vi "writeI32.vi"(8 "error in (no error)":errorcluster, 10 "Input":i32, 11 "ModbusBuffer in":refnum<class "ModbusBufferBuilder.lvclass">) -> (0 "error out":errorcluster, 3 "ModbusBuffer out":refnum<class "ModbusBufferBuilder.lvclass">)   [LabVIEW 2016, in "ModbusBufferBuilder.lvclass"]
uses:
  ModbusBufferBuilder.lvclass
  ModbusBufferBuilder.lvclass/ModbusBufferBuilder.ctl
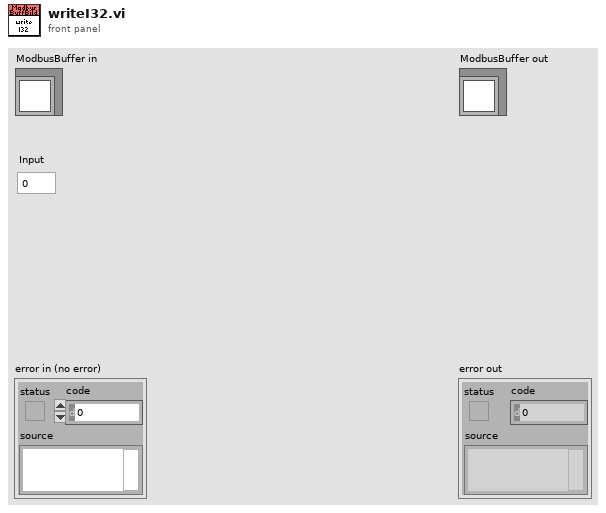
[diagram p1: front panel]
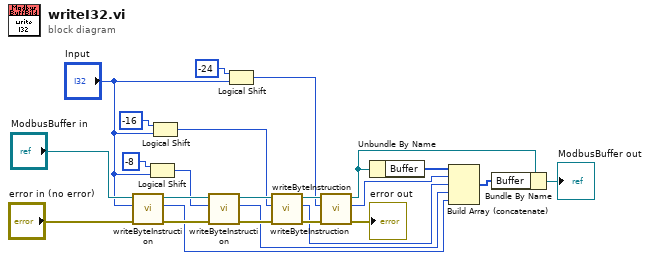
[diagram p0: block diagram]
diagram:
  n1 = call "writeByteInstruction.vi"("error in (no error)"="error in (no error)", "Input"="Input", "ModbusBuffer in"="ModbusBuffer in") -> ("error out"=w12:errorcluster, "Output"=w1:u16, "ModbusBuffer out"=w20:refnum<class "ModbusBufferBuilder.lvclass">)  [unwired: 6 in]
  n2 = Logical Shift(y=i16 -8, x="Input") -> (x << y=w16:i32)
  n3 = Logical Shift(y=i16 -16, x="Input") -> (x << y=w15:i32)
  n4 = call "writeByteInstruction.vi"("error in (no error)"=w12, "Input"=w16, "ModbusBuffer in"=w20) -> ("error out"=w11:errorcluster, "Output"=w2:u16, "ModbusBuffer out"=w19:refnum<class "ModbusBufferBuilder.lvclass">)  [unwired: 6 in]
  n5 = Logical Shift(y=i16 -24, x="Input") -> (x << y=w14:i32)
  n6 = call "writeByteInstruction.vi"("error in (no error)"=w11, "Input"=w15, "ModbusBuffer in"=w19) -> ("error out"=w10:errorcluster, "Output"=w3:u16, "ModbusBuffer out"=w18:refnum<class "ModbusBufferBuilder.lvclass">)  [unwired: 6 in]
  n7 = call "writeByteInstruction.vi"("error in (no error)"=w10, "Input"=w14, "ModbusBuffer in"=w18) -> ("error out"=→"error out":errorcluster, "Output"=w4:u16, "ModbusBuffer out"=w9:refnum<class "ModbusBufferBuilder.lvclass">)  [unwired: 6 in]
  n8 = Unbundle By Name(w9) -> ("Buffer"=w6:u16[])
  n9 = Build Array (concatenate)(w6, w4, w3, w2, w1) -> (w5:u16[])
  n10 = Bundle By Name(cluster=w9, "Buffer"=w5) -> (→"ModbusBuffer out":refnum<class "ModbusBufferBuilder.lvclass">)
